vi "Mem_ObtainQueue.vi"(8 "error in (no error)":errorcluster) -> (0 "error out":errorcluster, 3 "queue out":refnum<queue>)   [LabVIEW 2019, in "Memory Data Access.lvlib"]
uses:
  Memory Data Access.lvlib
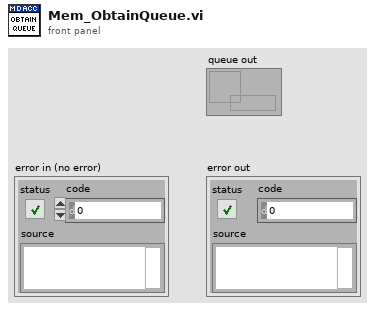
[diagram p1: front panel]
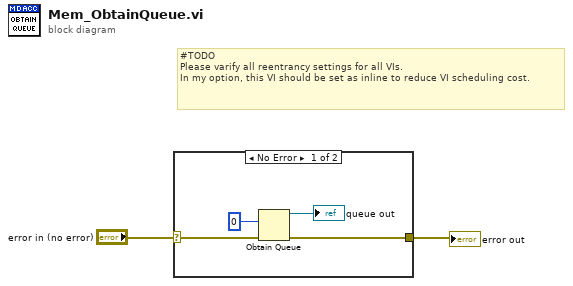
[diagram p0: block diagram]
diagram:
  # "#TODO\nPlease varify all reentrancy settings for all VIs.\nIn my option, this VI should be set as inline to reduce VI scheduling cost."
  n1 = case shown="No Error" "error in (no error)" {
    selector: "error in (no error)" -> [w3 w7]
    tunnel: [w4 w7] -> w2
    frame No Error {
      n2 = Obtain Queue(element data type=u64 0, error in (no error)=w3) -> (queue out=→"queue out":refnum<queue>, error out=w4:errorcluster)  [unwired: 3 in, 1 out]
    }
    frame Error {
    }
  }
  "error out" <- w2
